vi "BoP Model Control.vi"() -> ()   [LabVIEW 2017]
uses:
  <vilib>/Platform/TimedLoop/XDataNode/timing_clust.ctl
  <vilib>/Platform/TimedLoop/XDataNode/nitl_modes.ctl
  <vilib>/Platform/TimedLoop/XDataNode/wakeup.ctl
  <vilib>/Model Interface Toolkit/Model Interface Toolkit.lvclass/Model Interface Toolkit.ctl
  <vilib>/Model Interface Toolkit/Model Update.vi
  <vilib>/Model Interface Toolkit/Tick Model.vi
  <vilib>/Model Interface Toolkit/Probe Signals.vi
  <vilib>/Model Interface Toolkit/Multirate/Dispatch Model Tasks.vi
  <vilib>/Model Interface Toolkit/Call Model Start Routine.vi
  <vilib>/Model Interface Toolkit/Handle Error.vi
  <vilib>/Model Interface Toolkit/Multirate/Wait on Tasks.vi
  <vilib>/Model Interface Toolkit/Check Error.vi
  <vilib>/Model Interface Toolkit/Generate Error Cluster.vi
  <vilib>/Platform/TimedLoop/scheduler/LVUserAPI/Fire Software-Triggered Timing Source.vi
  <vilib>/Platform/TimedLoop/XDataNode/XDataNode.xnode
  <vilib>/Model Interface Toolkit/Model Interface Toolkit.lvclass
  <vilib>/Platform/TimedLoop/XDataNode/XDNodeRunTimeDep.lvlib
panel:
  in  "Stop":bool
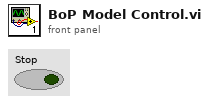
[diagram p1: front panel]
types:
  T1 = typedef "XDNodeRunTimeDep.lvlib/timing_clust.ctl" = cluster{"Expected End [f-1]":u64, "Actual End [f-1]":u64, "Finished Late? [f-1]":bool, "Expected End [i-1]":u64, "Actual End [i-1]":u64, "Finished Late? [i-1]":bool, "Expected Start [i]":u64, "Actual Start [i]":u64, "Expected Start [f]":u64, "Actual Start [f]":u64, "Source Name":string, "Structure Name":string, "Period":i64, "Deadline":i64, "Offset":i64, "Start":i64, "Priority":i32, "Timeout":i32, "Mode":T2, "Wakeup Reason":T3, "Error":errorcluster, "Source Type":string, "Secondary Source Type":string, "Global End Time":u64, "Global Start Time":u64, "Frame Duration":u64, "Iteration Duration":u64, "Assigned CPU":i32, "I/O Scan Engine Mode":u32}
  T2 = typedef "XDNodeRunTimeDep.lvlib/nitl_modes.ctl" = enum32{"No Change", "Process missed periods, maintain original phase", "Discard missed periods, maintain original phase", "Process missed periods, ignore original phase", "Discard missed periods, ignore original phase"}
  T3 = typedef "XDNodeRunTimeDep.lvlib/wakeup.ctl" = enum32{"Normal", "Aborted", "Asynchronous wakeup", "Timing source error", "Timed loop error", "Timeout"}
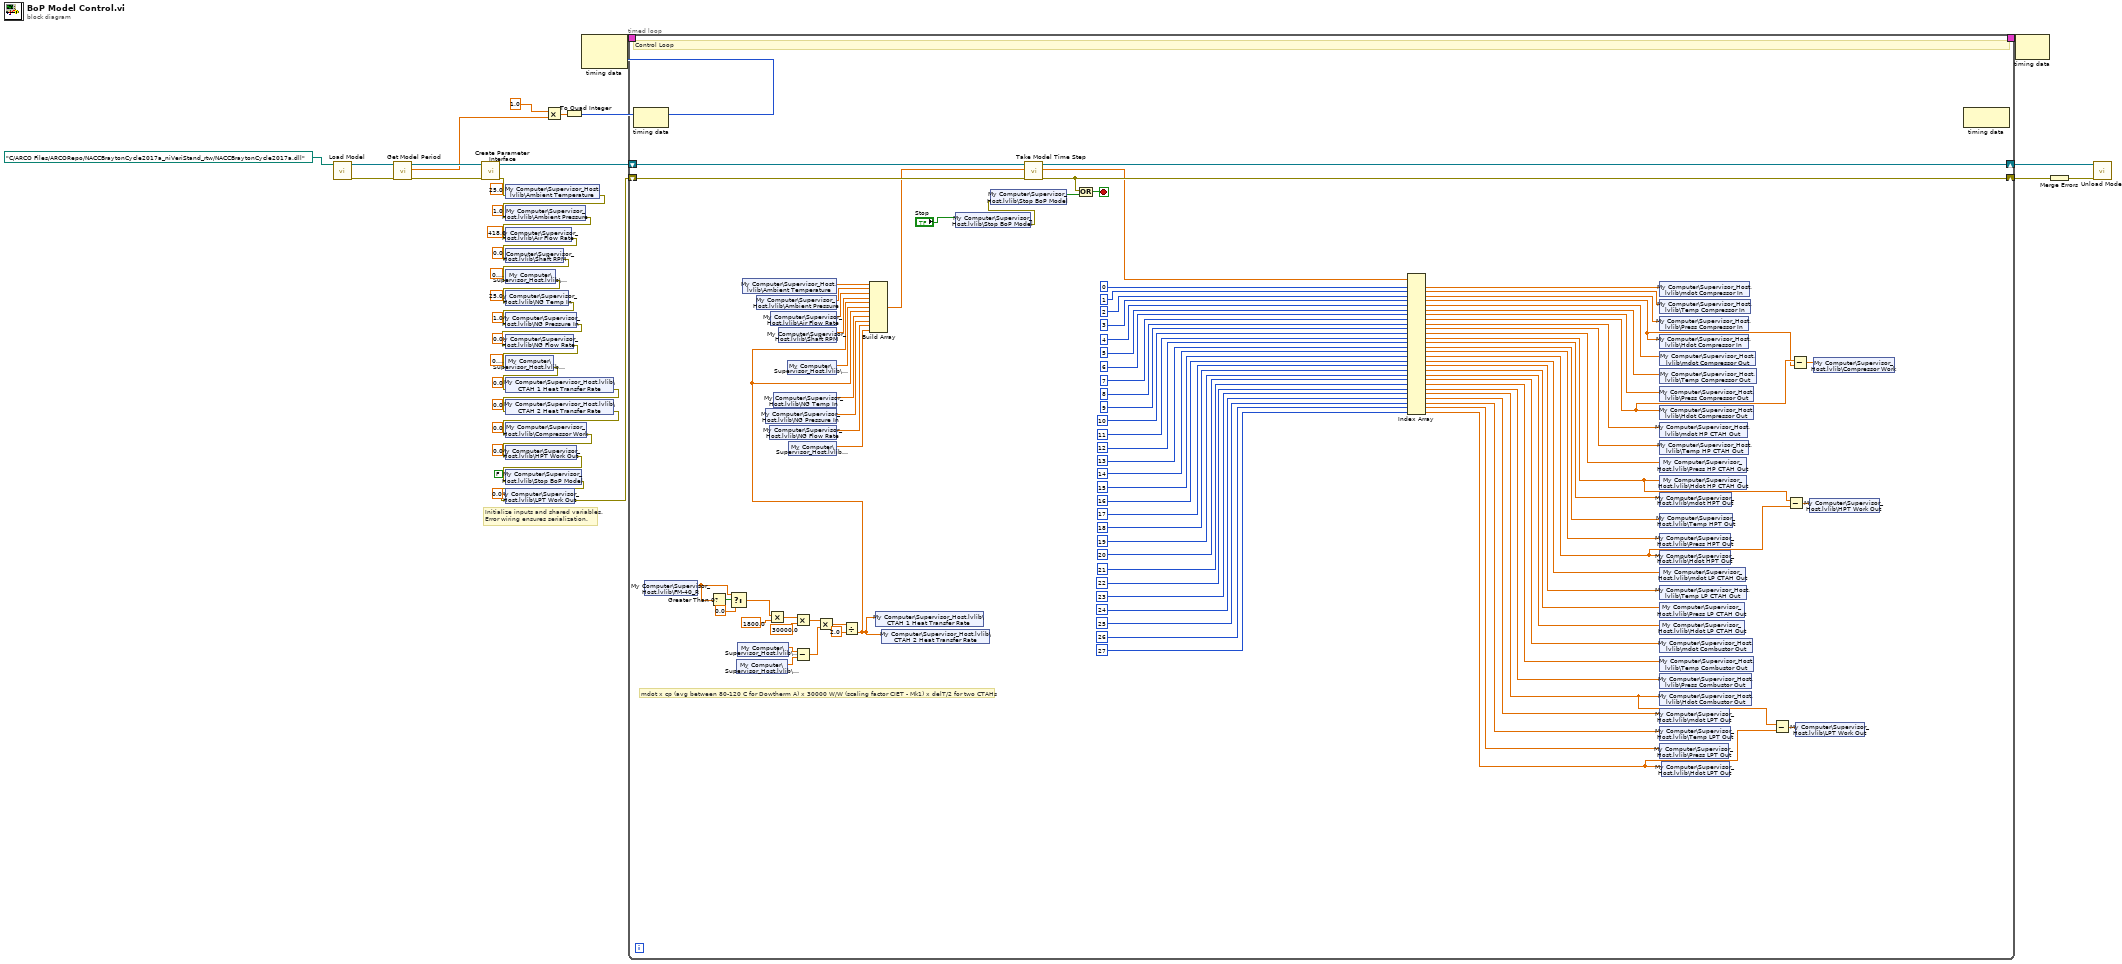
[diagram p0: block diagram]
diagram:
  # "Initialize inputs and shared variables.\nError wiring ensures serialization."
  n1 = call <vilib>:"Load Model.vi"("Model Path"=path "C:/ARCO Files/ARCORepo/NACCBraytonCycle2017a_niVeriStand_rtw/NACCBraytonCycle2017a.dll") -> ("error out"=w40:errorcluster, "Model out"=w43:refnum<class "Model Interface Toolkit.lvclass">)  [unwired: 9 in]
  n2 = call <vilib>:"Get Model Period.vi"("error in"=w40, "Model in"=w43) -> ("error out"=w39:errorcluster, "Model Period (s)"=w34:dbl, "Model out"=w42:refnum<class "Model Interface Toolkit.lvclass">)  [unwired: 7 in]
  n3 = call <vilib>:"Create Parameter Interface.vi"("error in"=w39, "Model in"=w42) -> ("error out"=w18:errorcluster, "Model out"=w41:refnum<class "Model Interface Toolkit.lvclass">)  [unwired: 7 in, 1 out]
  n4 = shared-variable "My Computer\\Supervisor_Host.lvlib\\Ambient Temperature"(sgl 25.0 ("Ambient Temperature"), error in=w18) -> (error out=w31:errorcluster)
  n5 = shared-variable "My Computer\\Supervisor_Host.lvlib\\Ambient Pressure"(sgl 1.0 ("Ambient Pressure"), error in=w31) -> (error out=w30:errorcluster)
  n6 = shared-variable "My Computer\\Supervisor_Host.lvlib\\Air Flow Rate"(sgl 418.0 ("Air Flow Rate"), error in=w30) -> (error out=w29:errorcluster)
  n7 = shared-variable "My Computer\\Supervisor_Host.lvlib\\Shaft RPM"(sgl 0.0 ("Shaft RPM"), error in=w29) -> (error out=w28:errorcluster)
  n8 = shared-variable "My Computer\\Supervisor_Host.lvlib\\HPT PR"(sgl 0.2 ("HPT PR"), error in=w28) -> (error out=w27:errorcluster)
  n9 = shared-variable "My Computer\\Supervisor_Host.lvlib\\NG Temp In"(sgl 25.0 ("NG Temp In"), error in=w27) -> (error out=w26:errorcluster)
  n10 = shared-variable "My Computer\\Supervisor_Host.lvlib\\NG Pressure In"(sgl 1.0 ("NG Pressure In"), error in=w26) -> (error out=w25:errorcluster)
  n11 = shared-variable "My Computer\\Supervisor_Host.lvlib\\NG Flow Rate"(sgl 0.0 ("NG Flow Rate"), error in=w25) -> (error out=w24:errorcluster)
  n12 = shared-variable "My Computer\\Supervisor_Host.lvlib\\LPT PR"(sgl 0.2 ("LPT PR"), error in=w24) -> (error out=w23:errorcluster)
  n13 = shared-variable "My Computer\\Supervisor_Host.lvlib\\CTAH 1 Heat Transfer Rate"(sgl 0.0 ("CTAH 1 Heat Transfer Rate"), error in=w23) -> (error out=w22:errorcluster)
  n14 = shared-variable "My Computer\\Supervisor_Host.lvlib\\CTAH 2 Heat Transfer Rate"(sgl 0.0 ("CTAH 2 Heat Transfer Rate"), error in=w22) -> (error out=w21:errorcluster)
  n15 = shared-variable "My Computer\\Supervisor_Host.lvlib\\Compressor Work"(sgl 0.0 ("Compressor Work"), error in=w21) -> (error out=w20:errorcluster)
  n16 = shared-variable "My Computer\\Supervisor_Host.lvlib\\HPT Work Out"(sgl 0.0 ("HPT Work Out"), error in=w20) -> (error out=w19:errorcluster)
  n17 = shared-variable "My Computer\\Supervisor_Host.lvlib\\Stop BoP Model"(FALSE ("Stop BoP Model"), error in=w19) -> (error out=w3:errorcluster)
  n18 = shared-variable "My Computer\\Supervisor_Host.lvlib\\LPT Work Out"(sgl 0.0 ("LPT Work Out"), error in=w3) -> (error out=w2:errorcluster)
  n19 = Multiply(x=1.0, y=w34) -> (x*y=w33:dbl)
  n20 = To Quad Integer(1:w33) -> (0:w32:i64)
  n21 = node-c288(w32) -> (w45:T1)  [unwired: 1 in]
  n22 = timed-loop {
    timing: w45 -> [_]
    timing-out: [_] -> w44
    shift-right: [w137] -> w38
    shift-left: w41 -> [w138]
    shift-right: [w134] -> w37
    shift-left: w2 -> [w136]
    stop <- w135 stop-if-true
    # "mdot x cp (avg between 80-120 C for Dowtherm A) x 30000 W/W (scaling factor CIET - Mk1) x delT/2 for two CTAHs"
    # "Control Loop"
    n23 = node-c288() -> ()  [unwired: 1 in, 1 out]
    n24 = shared-variable "My Computer\\Supervisor_Host.lvlib\\FM-40_R"() -> (w60:sgl)  [unwired: 1 in, 1 out]
    n25 = Greater Than 0?(x=w60) -> (x > 0?=w61:bool)
    n26 = Select(t=w60, s=w61, f=sgl 0.0) -> (s? t:f=w58:sgl)
    n27 = shared-variable "My Computer\\Supervisor_Host.lvlib\\BT-41_R"() -> (w65:sgl)  [unwired: 1 in, 1 out]
    n28 = shared-variable "My Computer\\Supervisor_Host.lvlib\\BT-43_R"() -> (w66:sgl)  [unwired: 1 in, 1 out]
    n29 = shared-variable "My Computer\\Supervisor_Host.lvlib\\Ambient Temperature"() -> (w131:sgl)  [unwired: 1 in, 1 out]
    n30 = shared-variable "My Computer\\Supervisor_Host.lvlib\\Ambient Pressure"() -> (w130:sgl)  [unwired: 1 in, 1 out]
    n31 = shared-variable "My Computer\\Supervisor_Host.lvlib\\NG Pressure In"() -> (w125:sgl)  [unwired: 1 in, 1 out]
    n32 = Multiply(x=w58, y=sgl 1800.0) -> (x*y=w69:sgl)
    n33 = shared-variable "My Computer\\Supervisor_Host.lvlib\\NG Flow Rate"() -> (w124:sgl)  [unwired: 1 in, 1 out]
    n34 = shared-variable "My Computer\\Supervisor_Host.lvlib\\Air Flow Rate"() -> (w129:sgl)  [unwired: 1 in, 1 out]
    n35 = shared-variable "My Computer\\Supervisor_Host.lvlib\\NG Temp In"() -> (w126:sgl)  [unwired: 1 in, 1 out]
    n36 = shared-variable "My Computer\\Supervisor_Host.lvlib\\Shaft RPM"() -> (w128:sgl)  [unwired: 1 in, 1 out]
    n37 = shared-variable "My Computer\\Supervisor_Host.lvlib\\HPT PR"() -> (w127:sgl)  [unwired: 1 in, 1 out]
    n38 = shared-variable "My Computer\\Supervisor_Host.lvlib\\LPT PR"() -> (w123:sgl)  [unwired: 1 in, 1 out]
    n39 = Multiply(x=w69, y=sgl 30000.0) -> (x*y=w67:sgl)
    n40 = Subtract(x=w66, y=w65) -> (x-y=w64:sgl)
    n41 = Multiply(x=w67, y=w64) -> (x*y=w63:sgl)
    n42 = Divide(x=w63, y=sgl 2.0) -> (x/y=w57:sgl)
    n43 = Build Array(w131, w130, w129, w128, w57, w127, w57, w126, w125, w124, w123) -> (w133:sgl[])
    n44 = shared-variable "My Computer\\Supervisor_Host.lvlib\\CTAH 1 Heat Transfer Rate"(w57) -> ()  [unwired: 1 in, 1 out]
    n45 = shared-variable "My Computer\\Supervisor_Host.lvlib\\CTAH 2 Heat Transfer Rate"(w57) -> ()  [unwired: 1 in, 1 out]
    n46 = shared-variable "My Computer\\Supervisor_Host.lvlib\\Stop BoP Model"("Stop") -> (error out=w47:errorcluster)  [unwired: 1 in]
    n47 = shared-variable "My Computer\\Supervisor_Host.lvlib\\Stop BoP Model"(error in=w47) -> (w72:bool)  [unwired: 1 out]
    n48 = call <vilib>:"Take Model Time Step.vi"("error in (no error)"=w136, "Inport Array"=w133, "Model in"=w138) -> ("error out"=w134:errorcluster, "Outport Array out"=w132:dbl[], "Model out"=w137:refnum<class "Model Interface Toolkit.lvclass">)  [unwired: 6 in]
    n49 = Or(x=w134, y=w72) -> (x .or. y?=w135:bool)
    n50 = Index Array(array=w132, index #1=0 ("index"), index #2=1 ("index"), index #3=2 ("index"), index #4=3 ("index"), index #5=4 ("index"), index #6=5 ("index"), index #7=6 ("index"), index #8=7 ("index"), index #9=8 ("index"), index #10=9 ("index"), index #11=10 ("index"), index #12=11 ("index"), index #13=12 ("index"), index #14=13 ("index"), index #15=14 ("index"), index #16=15 ("index"), index #17=16 ("index"), index #18=17 ("index"), index #19=18 ("index"), index #20=19 ("index"), index #21=20 ("index"), index #22=21 ("index"), index #23=22 ("index"), index #24=23 ("index"), index #25=24 ("index"), index #26=25 ("index"), index #27=26 ("index"), index #28=27 ("index")) -> (element #1=w94:dbl, element #2=w93:dbl, element #3=w92:dbl, element #4=w54:dbl, element #5=w91:dbl, element #6=w90:dbl, element #7=w89:dbl, element #8=w55:dbl, element #9=w88:dbl, element #10=w87:dbl, element #11=w86:dbl, element #12=w52:dbl, element #13=w85:dbl, element #14=w84:dbl, element #15=w83:dbl, element #16=w51:dbl, element #17=w82:dbl, element #18=w81:dbl, element #19=w80:dbl, element #20=w79:dbl, element #21=w78:dbl, element #22=w77:dbl, element #23=w76:dbl, element #24=w49:dbl, element #25=w75:dbl, element #26=w74:dbl, element #27=w73:dbl, element #28=w48:dbl)
    n51 = shared-variable "My Computer\\Supervisor_Host.lvlib\\mdot Compressor In"(w94) -> ()  [unwired: 1 in, 1 out]
    n52 = shared-variable "My Computer\\Supervisor_Host.lvlib\\Temp Compressor In"(w93) -> ()  [unwired: 1 in, 1 out]
    n53 = shared-variable "My Computer\\Supervisor_Host.lvlib\\Press Compressor In"(w92) -> ()  [unwired: 1 in, 1 out]
    n54 = shared-variable "My Computer\\Supervisor_Host.lvlib\\Hdot Compressor In"(w54) -> ()  [unwired: 1 in, 1 out]
    n55 = shared-variable "My Computer\\Supervisor_Host.lvlib\\mdot Compressor Out"(w91) -> ()  [unwired: 1 in, 1 out]
    n56 = shared-variable "My Computer\\Supervisor_Host.lvlib\\Temp Compressor Out"(w90) -> ()  [unwired: 1 in, 1 out]
    n57 = shared-variable "My Computer\\Supervisor_Host.lvlib\\Press Compressor Out"(w89) -> ()  [unwired: 1 in, 1 out]
    n58 = shared-variable "My Computer\\Supervisor_Host.lvlib\\Hdot Compressor Out"(w55) -> ()  [unwired: 1 in, 1 out]
    n59 = shared-variable "My Computer\\Supervisor_Host.lvlib\\mdot HP CTAH Out"(w88) -> ()  [unwired: 1 in, 1 out]
    n60 = shared-variable "My Computer\\Supervisor_Host.lvlib\\Temp HP CTAH Out"(w87) -> ()  [unwired: 1 in, 1 out]
    n61 = shared-variable "My Computer\\Supervisor_Host.lvlib\\Press HP CTAH Out"(w86) -> ()  [unwired: 1 in, 1 out]
    n62 = shared-variable "My Computer\\Supervisor_Host.lvlib\\Hdot HP CTAH Out"(w52) -> ()  [unwired: 1 in, 1 out]
    n63 = shared-variable "My Computer\\Supervisor_Host.lvlib\\mdot HPT Out"(w85) -> ()  [unwired: 1 in, 1 out]
    n64 = shared-variable "My Computer\\Supervisor_Host.lvlib\\Temp HPT Out"(w84) -> ()  [unwired: 1 in, 1 out]
    n65 = shared-variable "My Computer\\Supervisor_Host.lvlib\\Press HPT Out"(w83) -> ()  [unwired: 1 in, 1 out]
    n66 = shared-variable "My Computer\\Supervisor_Host.lvlib\\Hdot HPT Out"(w51) -> ()  [unwired: 1 in, 1 out]
    n67 = shared-variable "My Computer\\Supervisor_Host.lvlib\\mdot LP CTAH Out"(w82) -> ()  [unwired: 1 in, 1 out]
    n68 = shared-variable "My Computer\\Supervisor_Host.lvlib\\Temp LP CTAH Out"(w81) -> ()  [unwired: 1 in, 1 out]
    n69 = shared-variable "My Computer\\Supervisor_Host.lvlib\\Press LP CTAH Out"(w80) -> ()  [unwired: 1 in, 1 out]
    n70 = shared-variable "My Computer\\Supervisor_Host.lvlib\\Hdot LP CTAH Out"(w79) -> ()  [unwired: 1 in, 1 out]
    n71 = shared-variable "My Computer\\Supervisor_Host.lvlib\\mdot Combustor Out"(w78) -> ()  [unwired: 1 in, 1 out]
    n72 = shared-variable "My Computer\\Supervisor_Host.lvlib\\Temp Combustor Out"(w77) -> ()  [unwired: 1 in, 1 out]
    n73 = shared-variable "My Computer\\Supervisor_Host.lvlib\\Press Combustor Out"(w76) -> ()  [unwired: 1 in, 1 out]
    n74 = shared-variable "My Computer\\Supervisor_Host.lvlib\\Hdot Combustor Out"(w49) -> ()  [unwired: 1 in, 1 out]
    n75 = shared-variable "My Computer\\Supervisor_Host.lvlib\\mdot LPT Out"(w75) -> ()  [unwired: 1 in, 1 out]
    n76 = shared-variable "My Computer\\Supervisor_Host.lvlib\\Temp LPT Out"(w74) -> ()  [unwired: 1 in, 1 out]
    n77 = shared-variable "My Computer\\Supervisor_Host.lvlib\\Press LPT Out"(w73) -> ()  [unwired: 1 in, 1 out]
    n78 = shared-variable "My Computer\\Supervisor_Host.lvlib\\Hdot LPT Out"(w48) -> ()  [unwired: 1 in, 1 out]
    n79 = Subtract(x=w49, y=w48) -> (x-y=w50:dbl)
    n80 = Subtract(x=w52, y=w51) -> (x-y=w53:dbl)
    n81 = Subtract(x=w55, y=w54) -> (x-y=w56:dbl)
    n82 = shared-variable "My Computer\\Supervisor_Host.lvlib\\LPT Work Out"(w50) -> ()  [unwired: 1 in, 1 out]
    n83 = shared-variable "My Computer\\Supervisor_Host.lvlib\\HPT Work Out"(w53) -> ()  [unwired: 1 in, 1 out]
    n84 = shared-variable "My Computer\\Supervisor_Host.lvlib\\Compressor Work"(w56) -> ()  [unwired: 1 in, 1 out]
    n85 = node-c288() -> ()  [unwired: 1 in, 1 out]
  }
  n86 = node-c288(w44) -> ()  [unwired: 1 out]
  n87 = Merge Errors(w37) -> (w36:errorcluster)
  n88 = call <vilib>:"Unload Model.vi"("error in (no error)"=w36, "Model in"=w38) -> ()  [unwired: 9 in, 1 out]
